vi "Unsubscribe.vi"(6 "timeout (1000 ms)":i32=1000, 8 "error in (no error)":errorcluster, 9 "Packet ID (empty: Generate new)":u16 format="%04x", 10 "Topics":string[](array[string]), 11 "MQTT_Base in":refnum<class "MQTT_Base.lvclass">) -> (0 "error out":errorcluster, 1 "UNSUBACK Packet ID":u16 format="%04x", 3 "MQTT_Base out":refnum<class "MQTT_Base.lvclass">)   [LabVIEW 2013, in "MQTT Server.lvlib" / "MQTT_Base.lvclass"]
uses:
  MQTT_Base.lvclass
  Control Packets/ControlPacket/ControlPacket.lvclass/ControlPacket.ctl
  Control Packets/UNSUBSCRIBE/UNSUBSCRIBE.lvclass
  Control Packets/ControlPacket/ControlPacket.lvclass
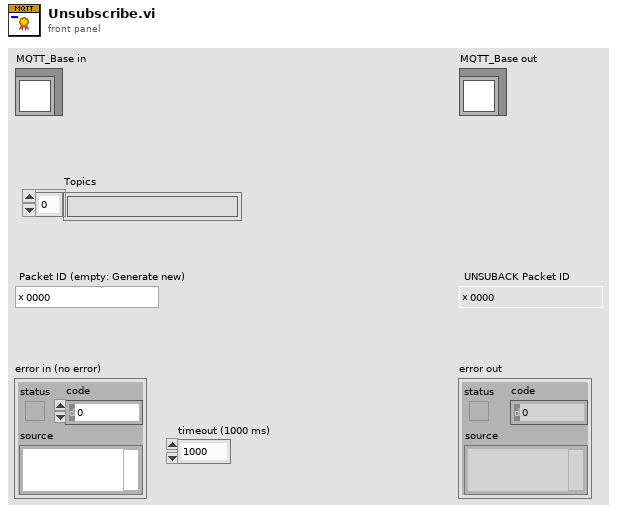
[diagram p1: front panel]
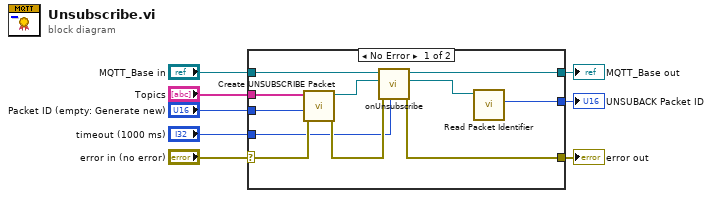
[diagram p0: block diagram]
diagram:
  n1 = case shown="No Error" "error in (no error)" {
    selector: "error in (no error)" -> [w18 w21]
    tunnel: [w13 w21] -> w7
    tunnel: [w16 w20] -> w5
    tunnel: "MQTT_Base in" -> [w17 w20]
    tunnel: "Topics" -> [w19 _]
    tunnel: "Packet ID (empty: Generate new)" -> [w12 _]
    tunnel: [w11 _] -> w2
    tunnel: "timeout (1000 ms)" -> [w9 _]
    frame No Error {
      n2 = call "Create UNSUBSCRIBE Packet.vi"("error in (no error)"=w18, "Packet ID (0: generate new)"=w12, "Topic Subscriptions"=w19) -> ("error out"=w14:errorcluster, "UNSUBSCRIBE out"=w15:refnum<class "UNSUBSCRIBE.lvclass">)  [unwired: 7 in]
      n3 = call-dynamic "onUnsubscribe.vi"("timeout (0ms : no ack)"=w9, "error in (no error)"=w14, "UNSUBSCRIBE"=w15, "MQTT_Base in"=w17) -> ("error out"=w13:errorcluster, "UNSUBACK"=w10:refnum<class "UNSUBACK.lvclass">, "MQTT_Base out"=w16:refnum<class "MQTT_Base.lvclass">)  [unwired: 5 in]
      n4 = call "Read Packet Identifier.vi"("ControlPacket in"=w10) -> ("Packet Identifier"=w11:u16)  [unwired: 9 in, 1 out]
    }
    frame Error {
    }
  }
  "error out" <- w7
  "MQTT_Base out" <- w5
  "UNSUBACK Packet ID" <- w2
